vi "tsapp_transmit_lin_async.vi"(8 "error in (no error)":errorcluster, 10 "LIN_Transmit":T1 {"Channel" items=["CHN1", "CHN2", "CHN3", "CHN4", "CHN5", "CHN6", "CHN7", "CHN8", "CHN9", "CHN10", "CHN11", "CHN12", "CHN13", "CHN14", "CHN15", "CHN16", "CHN17", "CHN18", "CHN19", "CHN20", "CHN21", "CHN22", "CHN23", "CHN24", "CHN25", "CHN26", "CHN27", "CHN28", "CHN29", "CHN30", "CHN31", "CHN32"]; "ID" format="%.0x"; "DLC" format="%.0x"; "Set_node_funtiontype" items=["MasterNode", "SlaveNode", "MonitorNote"]}, 11 "Path":path) -> (0 "error out":errorcluster, 2 "return":i32, 3 "Path output":path)   [LabVIEW 2014]
doc: "Function Introduction :\nAsynchronous sending of LIN messages\nCall location :\nIn situations where LIN messages need to be sent\ninput parameter :\nALIN: LIN message data\nReturn value :\n==0: Sent successfully\nOther values: Sending failed"
uses:
  Typedef/TLibLIN.ctl
  Typedef/TSLIN_Transmit.ctl
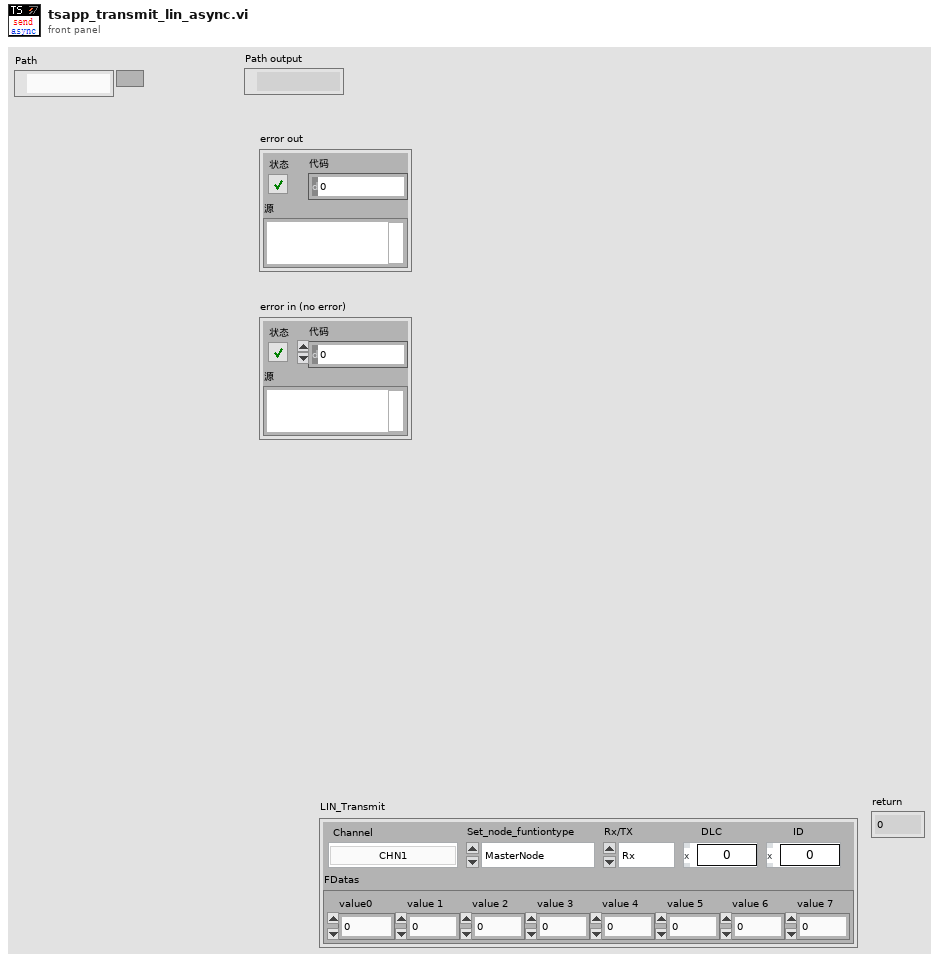
[diagram p1: front panel]
types:
  T1 = typedef "TSLIN_Transmit.ctl" = cluster{"Channel":i32, "Rx/TX":enum16{"Rx", "Tx"}, "Set_node_funtiontype":i32, "DLC":u32, "ID":u32, "FDatas":cluster{"value0":u8, "value 1":u8, "value 2":u8, "value 3":u8, "value 4":u8, "value 5":u8, "value 6":u8, "value 7":u8}}
  T2 = typedef "TLibLIN.ctl" = cluster{"Ch":u8, "Code":u8, "Properties":u8, "FDLC":u8, "ID":u8, "Checksum":u8, "FStaus":u8, "FTimeUS":u64, "FDatas":cluster{"value0":u8, "value 1":u8, "value 2":u8, "value 3":u8, "value 4":u8, "value 5":u8, "value 6":u8, "value 7":u8}}
  T3 = cluster{"value0":u8, "value 1":u8, "value 2":u8, "value 3":u8, "value 4":u8, "value 5":u8, "value 6":u8, "value 7":u8}
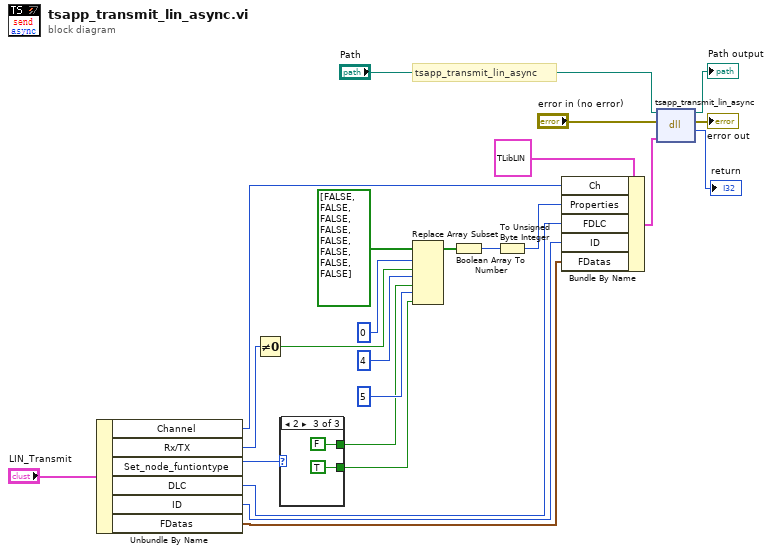
[diagram p0: block diagram]
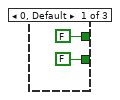
[diagram p2: hidden frame]
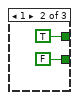
[diagram p3: hidden frame]
diagram:
  # "tsapp_transmit_lin_async"
  n1 = Unbundle By Name("LIN_Transmit") -> ("Channel"=w13:i32, "Rx/TX"=w10:enum16{"Rx", "Tx"}, "Set_node_funtiontype"=w6:i32, "DLC"=w12:u32, "ID"=w2:u32, "FDatas"=w1:T3)
  n2 = Not Equal To 0?(x=w10) -> (x != 0?=w9:bool)
  n3 = case shown="2" w6 {
    tunnel: [FALSE TRUE FALSE] -> w5
    tunnel: [FALSE FALSE TRUE] -> w4
    frame 0, Default {
    }
    frame 1 {
    }
    frame 2 {
    }
  }
  n4 = Replace Array Subset(array=bool[] [FALSE, FALSE, FALSE, FALSE, FALSE, FALSE, FALSE, FALSE], new element #1=w9, index #1=0 ("索引"), new element #2=w5, index #2=4 ("索引"), new element #3=w4, index #3=5 ("索引")) -> (w17:bool[])
  n5 = Boolean Array To Number(Boolean array=w17) -> (number=w16:u32)
  n6 = To Unsigned Byte Integer(number=w16) -> (unsigned 8bit integer=w15:u8)
  n7 = Bundle By Name(cluster=T2 {"Ch"=0, "Code"=0, "Properties"=0, "FDLC"=0, "ID"=0, "Checksum"=0, "FStaus"=0, "FTimeUS"=0, "FDatas"={"value0"=0, "value 1"=0, "value 2"=0, "value 3"=0, "value 4"=0, "value 5"=0, "value 6"=0, "value 7"=0}} ("TLIBLIN"), "Ch"=w13, "Properties"=w15, "FDLC"=w12, "ID"=w2, "FDatas"=w1) -> (w20:T2)
  n8 = dll-call lib="PTH2@abs EDemo同星TSCAN_V1.4_20220301ConfigTSMaster.dll" fn="tsapp_transmit_lin_async"(path in="Path", error in="error in (no error)", "LINDATA"=w20) -> (path out=→"Path output":path, error out=→"error out":errorcluster, "tsapp_transmit_can_async"=→"return":i32)  [unwired: 2 in]
